vi "LED_randwait.vi"() -> ()   [LabVIEW 2012]
uses:
  <vilib>/rvi/Emulation/niFpgaSctlEmulationGetInTimedLoop.vi
  <vilib>/rvi/Emulation/niFpgaSctlEmulationGlobalWrite.vi
  <vilib>/rvi/eio/common/nirviEmuTemplateMethod_errors.vi
  <vilib>/eio/EIONode/EIONode.xnode
panel:
  in  "reset":bool
  in  "FPGA I/O In":refnum<k21>="IO Module\\D0 0"
  out "Total number of pulses sent":u64
  out "Is Test Pulse?":bool
  in  "Testpulse Time Delay (20 ns ticks)":u32=15
  in  "Testpulser On/Off":bool
  in  "Testpulse duration (20 ns ticks)":u32=1
  in  "Randomly generated testpulse separation input (20 ns ticks)":u32=50000
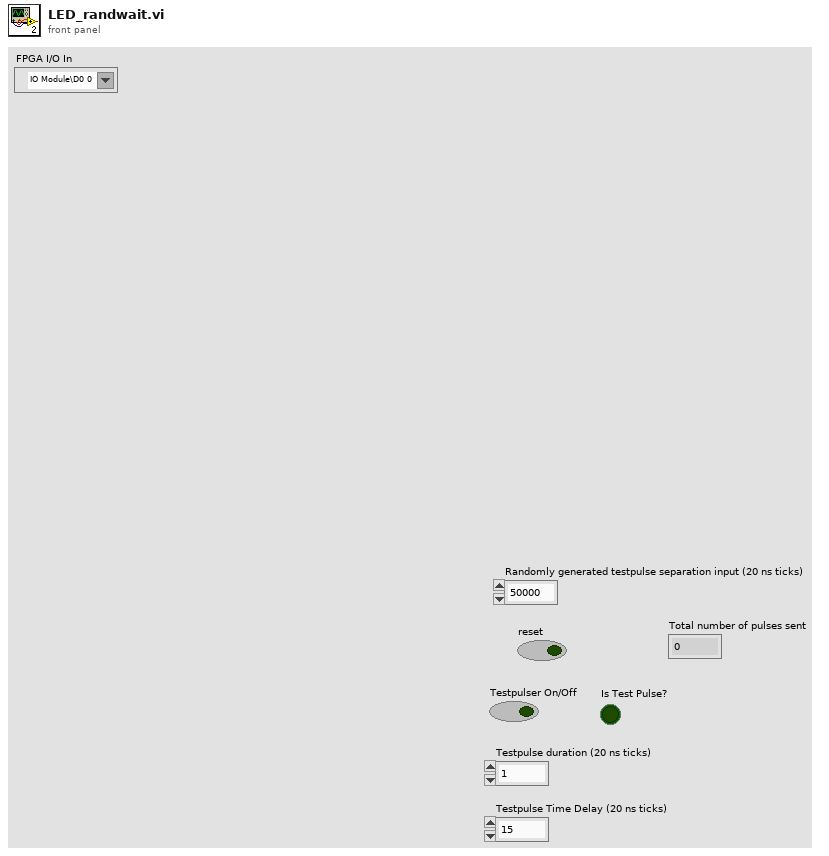
[diagram p1: front panel]
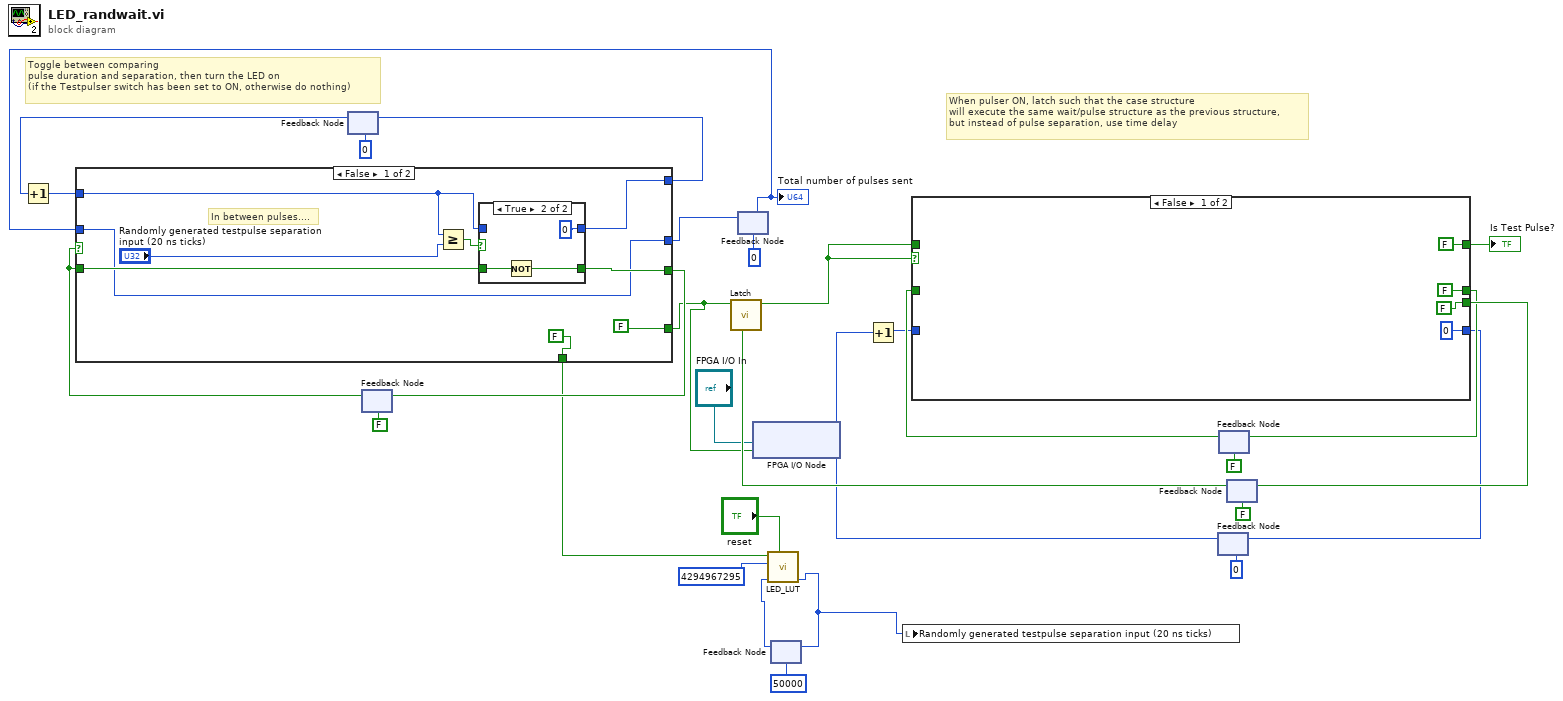
[diagram p0: block diagram]
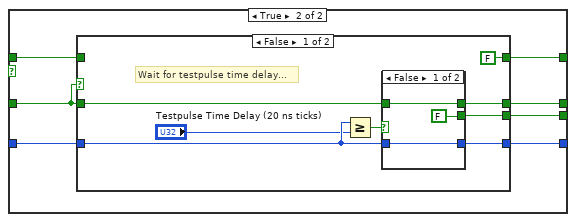
[diagram p2: hidden frame]
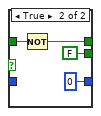
[diagram p3: hidden frame]
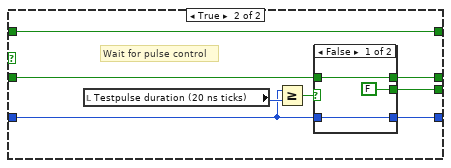
[diagram p4: hidden frame]
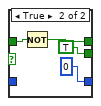
[diagram p5: hidden frame]
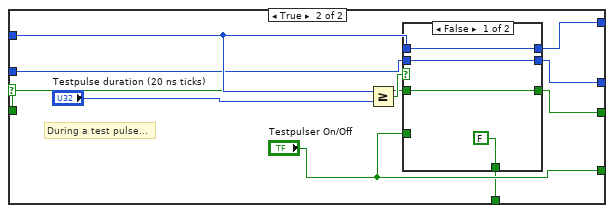
[diagram p7: hidden frame]
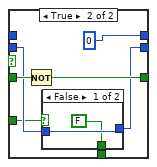
[diagram p8: hidden frame]
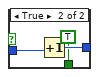
[diagram p9: hidden frame]
diagram:
  # "Toggle between comparing \npulse duration and separation, then turn the LED on\n(if the Testpulser switch has been set to ON, otherwise do nothing)"
  # "When pulser ON, latch such that the case structure\nwill execute the same wait/pulse structure as the previous structure, \nbut instead of pulse separation, use time delay"
  n1 = feedback #1(u32 0) -> (w16:u32)
  n2 = Increment(x=w16) -> (x+1=w13:u32)
  n3 = feedback #2(FALSE) -> (w19:bool)
  n4 = feedback #3(u64 0) -> (w11:u64)
  "Total number of pulses sent" <- w11
  n5 = case shown="False" w19 {
    tunnel: w13 -> [w36 w52]
    tunnel: [w39 w53] -> w17
    tunnel: [w38 w54] -> w6
    tunnel: [FALSE ("IO Module\\D0 0") "Testpulser On/Off"] -> w2
    tunnel: w19 -> [w34 w49]
    tunnel: w11 -> [w33 w48]
    tunnel: [w33 w47] -> w12
    tunnel: [FALSE ("IO Module\\D0 0") w45] -> w1
    frame False {
      # "In between pulses...."
      n6 = Greater Or Equal?(x=w36, y="Randomly generated testpulse separation input (20 ns ticks)") -> (x >= y?=w35:bool)
      n7 = case shown="True" w35 {
        tunnel: [w41 u32 0] -> w39
        tunnel: w36 -> [w41 _]
        tunnel: [w40 w43] -> w38
        tunnel: w34 -> [w40 w42]
        frame False {
        }
        frame True {
          n8 = Not(x=w42) -> (.not. x?=w43:bool)
        }
      }
    }
    frame True {
      # "During a test pulse..."
      n9 = Greater Or Equal?(x=w52, y="Testpulse duration (20 ns ticks)") -> (x >= y?=w51:bool)
      n10 = case shown="False" w51 {
        tunnel: w52 -> [w58 _]
        tunnel: [w57 w65] -> w54
        tunnel: [w58 u32 0] -> w53
        tunnel: w49 -> [w57 w63]
        tunnel: w48 -> [w56 w62]
        tunnel: [w56 w61] -> w47
        tunnel: "Testpulser On/Off" -> [_ w60]
        tunnel: [FALSE w59] -> w45
        frame False {
        }
        frame True {
          n11 = Not(x=w63) -> (.not. x?=w65:bool)
          n12 = case shown="False" w60 {
            tunnel: w62 -> [w67 w70]
            tunnel: [w67 w69] -> w61
            tunnel: [FALSE TRUE] -> w59
            frame False {
            }
            frame True {
              n13 = Increment(x=w70) -> (x+1=w69:u64)
            }
          }
        }
      }
    }
  }
  n14 = feedback-in #1(w17) -> ()
  n15 = feedback-in #2(w6) -> ()
  n16 = feedback-in #3(w12) -> ()
  n17 = xnode "FPGA I/O Node"("I/O Item"=w2, "FPGA I/O In"="FPGA I/O In") -> ()  [unwired: 1 out]
  n18 = feedback #4(u32 50000 ("Randomly generated testpulse separation out")) -> (w5:u32)
  n19 = call "LED_LUT.vi"("reset"="reset", "Previous value of randomly generated testpulse separation"=w5, "seed"=u32 4294967295, "Need a new random number?"=w1) -> ("Randomly generated testpulse separation out"=w4:u32)  [unwired: 7 in]
  n20 = feedback-in #4(w4) -> ()
  n21 = local write "Randomly generated testpulse separation input (20 ns ticks)"(w4) -> ()
  n22 = feedback #5(u32 0) -> (w21:u32)
  n23 = Increment(x=w21) -> (x+1=w22:u32)
  n24 = feedback #6(FALSE) -> (w25:bool)
  n25 = feedback #7(FALSE) -> (w29:bool)
  n26 = call "Latch.vi"("Reset"=w29, "Input"=w2) -> ("Output"=w30:bool)  [unwired: 9 in]
  n27 = case shown="False" w30 {
    tunnel: w30 -> [_ w76]
    tunnel: [FALSE w78] -> w14
    tunnel: w22 -> [_ w79]
    tunnel: [u32 0 w77] -> w23
    tunnel: w25 -> [_ w81]
    tunnel: [FALSE w80] -> w26
    tunnel: [FALSE w75] -> w28
    frame False {
    }
    frame True {
      n28 = case shown="False" w81 {
        tunnel: w81 -> [w88 w101]
        tunnel: [w87 w100] -> w80
        tunnel: w79 -> [w84 w102]
        tunnel: [FALSE w98] -> w78
        tunnel: [w85 w99] -> w77
        tunnel: w76 -> [_ w98]
        tunnel: [w82 w97] -> w75
        frame False {
          # "Wait for testpulse time delay..."
          n29 = Greater Or Equal?(x=w84, y="Testpulse Time Delay (20 ns ticks)") -> (x >= y?=w89:bool)
          n30 = case shown="False" w89 {
            tunnel: w88 -> [w92 w96]
            tunnel: [w92 w95] -> w87
            tunnel: [w91 u32 0] -> w85
            tunnel: w84 -> [w91 _]
            tunnel: [FALSE FALSE] -> w82
            frame False {
            }
            frame True {
              n31 = Not(x=w96) -> (.not. x?=w95:bool)
            }
          }
        }
        frame True {
          # "Wait for pulse control"
          n32 = local read "Testpulse duration (20 ns ticks)"() -> (w104:u32)
          n33 = Greater Or Equal?(x=w102, y=w104) -> (x >= y?=w103:bool)
          n34 = case shown="False" w103 {
            tunnel: w102 -> [w106 _]
            tunnel: w101 -> [w107 w110]
            tunnel: [w107 w109] -> w100
            tunnel: [w106 u32 0] -> w99
            tunnel: [FALSE TRUE] -> w97
            frame False {
            }
            frame True {
              n35 = Not(x=w110) -> (.not. x?=w109:bool)
            }
          }
        }
      }
    }
  }
  "Is Test Pulse?" <- w14
  n36 = feedback-in #5(w23) -> ()
  n37 = feedback-in #6(w26) -> ()
  n38 = feedback-in #7(w28) -> ()
